vi "field_sweep_agilent.vi"() -> ()   [LabVIEW 2017]
uses:
  Controls/State.ctl
  Controls/Data.ctl
  Controls/Instruments.ctl
  <vilib>/Utility/error.llb/DialogType.ctl
  <vilib>/DAQmx/write.llb/DAQmx Write (Analog DBL 1Chan 1Samp).vi
  <vilib>/DAQmx/create/channels.llb/DAQmx Create Channel (AO-Voltage-Basic).vi
  <vilib>/DAQmx/miscellaneous.llb/DAQmx Fill In Error Info.vi
  <instrlib>/LakeShore 336/Public/Data/Sensor Data (Single Reading).vi
  <instrlib>/Keysight PNA Series/Keysight PNA Series.lvlib
  <instrlib>/LakeShore 336/Lake Shore 336.lvlib
panel:
  in  "Start Over flag":bool
  out "Temp. Contr. Name (out)":refnum<visa-resource-name>
  in  "Temp. Contr. Name (in)":refnum<visa-resource-name>="LakeShore336"
  out "VNA name (out)":refnum<visa-resource-name>
  in  "VNA name (in)":refnum<visa-resource-name>="vna"
  in  "Display Format":i32(ring) items=["Magnitude Linear", "Magnitude Logarithmic", "Phase", "Unwrapped phase", "Imaginary", "Real", "Polar", "Smith Chart", "Smith Admittance", "SWR", "Group Delay", "Kelvin", "Fahrenheit", "Celsius"]
  in  "Data Type":i32(ring) items=["FDATA", "RDATA", "SDATA", "FMEM", "SMEM", "SDIV"]
  in  "Sweep Generation":i32(ring)=1 items=["Stepped", "Analog"]
  in  "Sweep Mode":i32(ring) items=["Chopped", "Alternate"]
  in  "Sweep Type":i32(ring) items=["Linear", "Logarithmic", "Power", "CW", "Segment", "Phase"]
  out "Gaussmeter Name (out)":refnum<visa-resource-name>
  in  "Gaussmeter Name (in)":refnum<visa-resource-name>="Lakeshore_475"
  in  "Clear button":bool
  in  "Hysteresis":bool caption="Hysteresis On/Off"
  out "DAQ channel (out)":tag="DAQ_6363/ao1"
  in  "Averaging Points":i32=10 min=1 max=3201 step=1
  in  "DAQ channel (in)":tag="DAQ_6363/ao1"
  in  "Exit Button":bool
  in  "IF Bandwidth":dbl(ring)=300.0 items=["10 Hz"=10.0, "30 Hz"=30.0, "100 Hz"=100.0, "300 Hz"=300.0, "1 KHz"=1000.0, "3 KHz"=3000.0, "10 KHz"=10000.0, "30 KHz"=30000.0]
  in  "Speed (Oe/sec)":dbl=50.0
  in  "Frequency (Hz)":dbl=4550000000.0 min=10000000.0 max=6000000000.0
  in  "Save Button":bool
  out "Status":string="Initializing..."
  out "Cursor":cluster{"x":dbl, "y":dbl} {"x" format="%.2f"; "y" format="%.5f"}
  out "Error Out":errorcluster={"status"=TRUE, "code"=-1073807346, "source"="VISA Open in Keysight PNA Series.lvlib:Initialize.vi->field_sweep_agilent.vi"}
  in  "Error In (no error)":errorcluster
  out "SpectrumGraph":cluster{"Old Field":dbl[], "Old Signal":dbl[]}[](graph)
  in  "S-parameter":i32(ring) caption="Measurement" items=["S11", "S21"]
  in  "Start Button":bool
  in  "Stop Button":bool
  in  "Output Power (dBm)":dbl=1.0 min=-25.0 max=5.0 step=0.5
  in  "Number of Points":i32=2000 min=1 max=3201 step=1
  in  "Stop H Field (Oe)":dbl=4200.0 min=-6000.0 max=6000.0 format="%#_6f"
  in  "Start H Field (Oe)":dbl=25.0 min=-6000.0 max=6000.0 format="%#_6f"
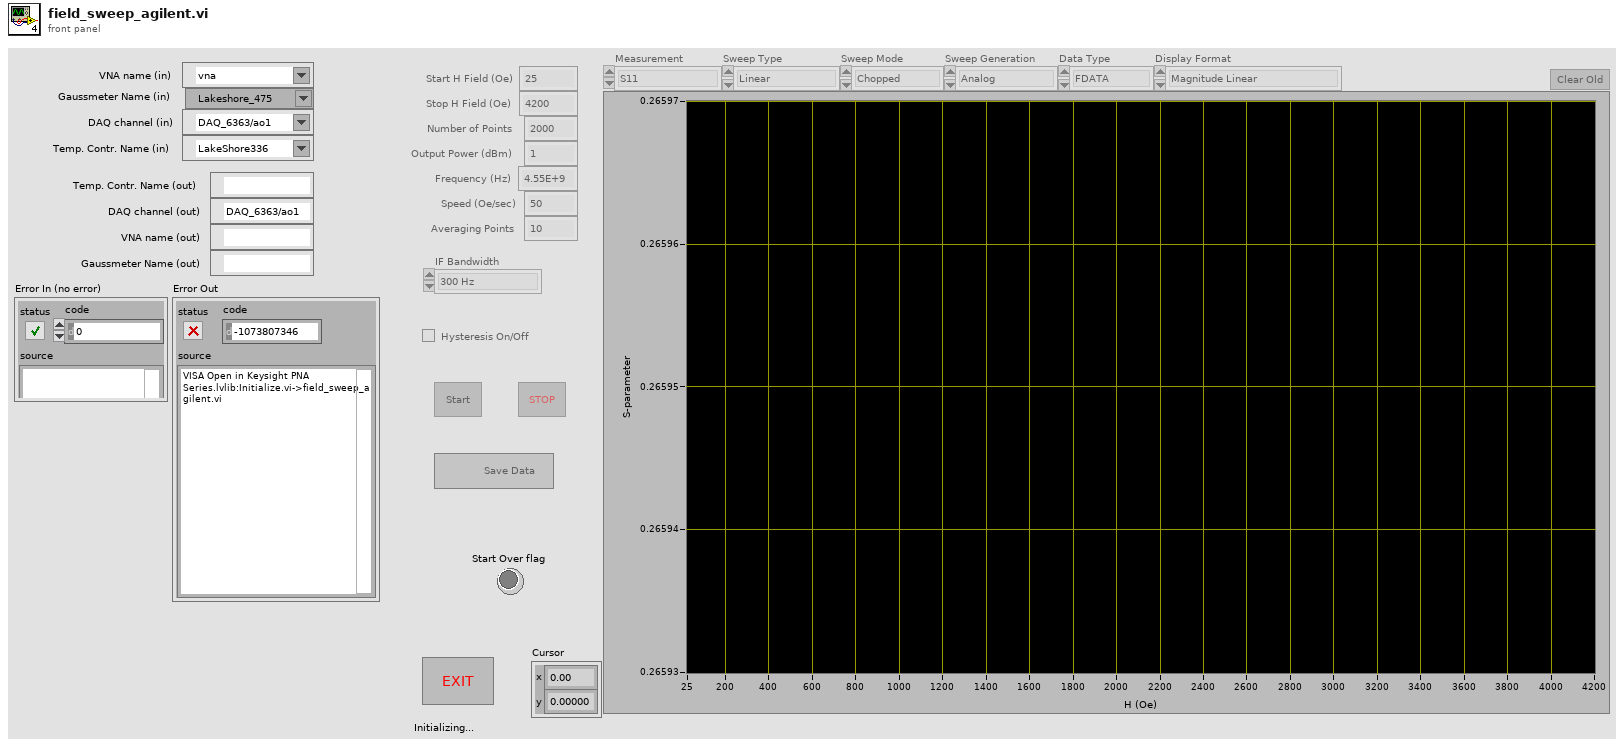
[diagram p1: front panel]
types:
  T1 = typedef "Instruments.ctl" = cluster{"Gaussmeter Name":refnum<visa-resource-name>, "VNA name":refnum<visa-resource-name>, "DAQ channel":tag, "DAQ task":refnum<k21>, "Temp. Contr. Name":refnum<visa-resource-name>}
  T2 = typedef "Data.ctl" = cluster{"Field":dbl[], "Signal":dbl[], "Temperature":dbl[], "Old Field":dbl[], "Old Signal":dbl[], "Old Temperature":dbl[]}
  T3 = typedef "State.ctl" = enum16{"Init", "Idle", "Sweeping up", "Sweeping down", "Running", "Running first time", "Running down", "Shutdown"}
  T4 = cluster{"Baud Rate":u32, "Parity":u16, "Data Bits":u16, "Stop Bits":u16, "Flow Control":u16}
  T5 = typedef "DialogType.ctl" = u16
  T6 = typedef "LVPoint32TypeDef.ctl" = cluster{"Horizontal":i32, "Vertical":i32}
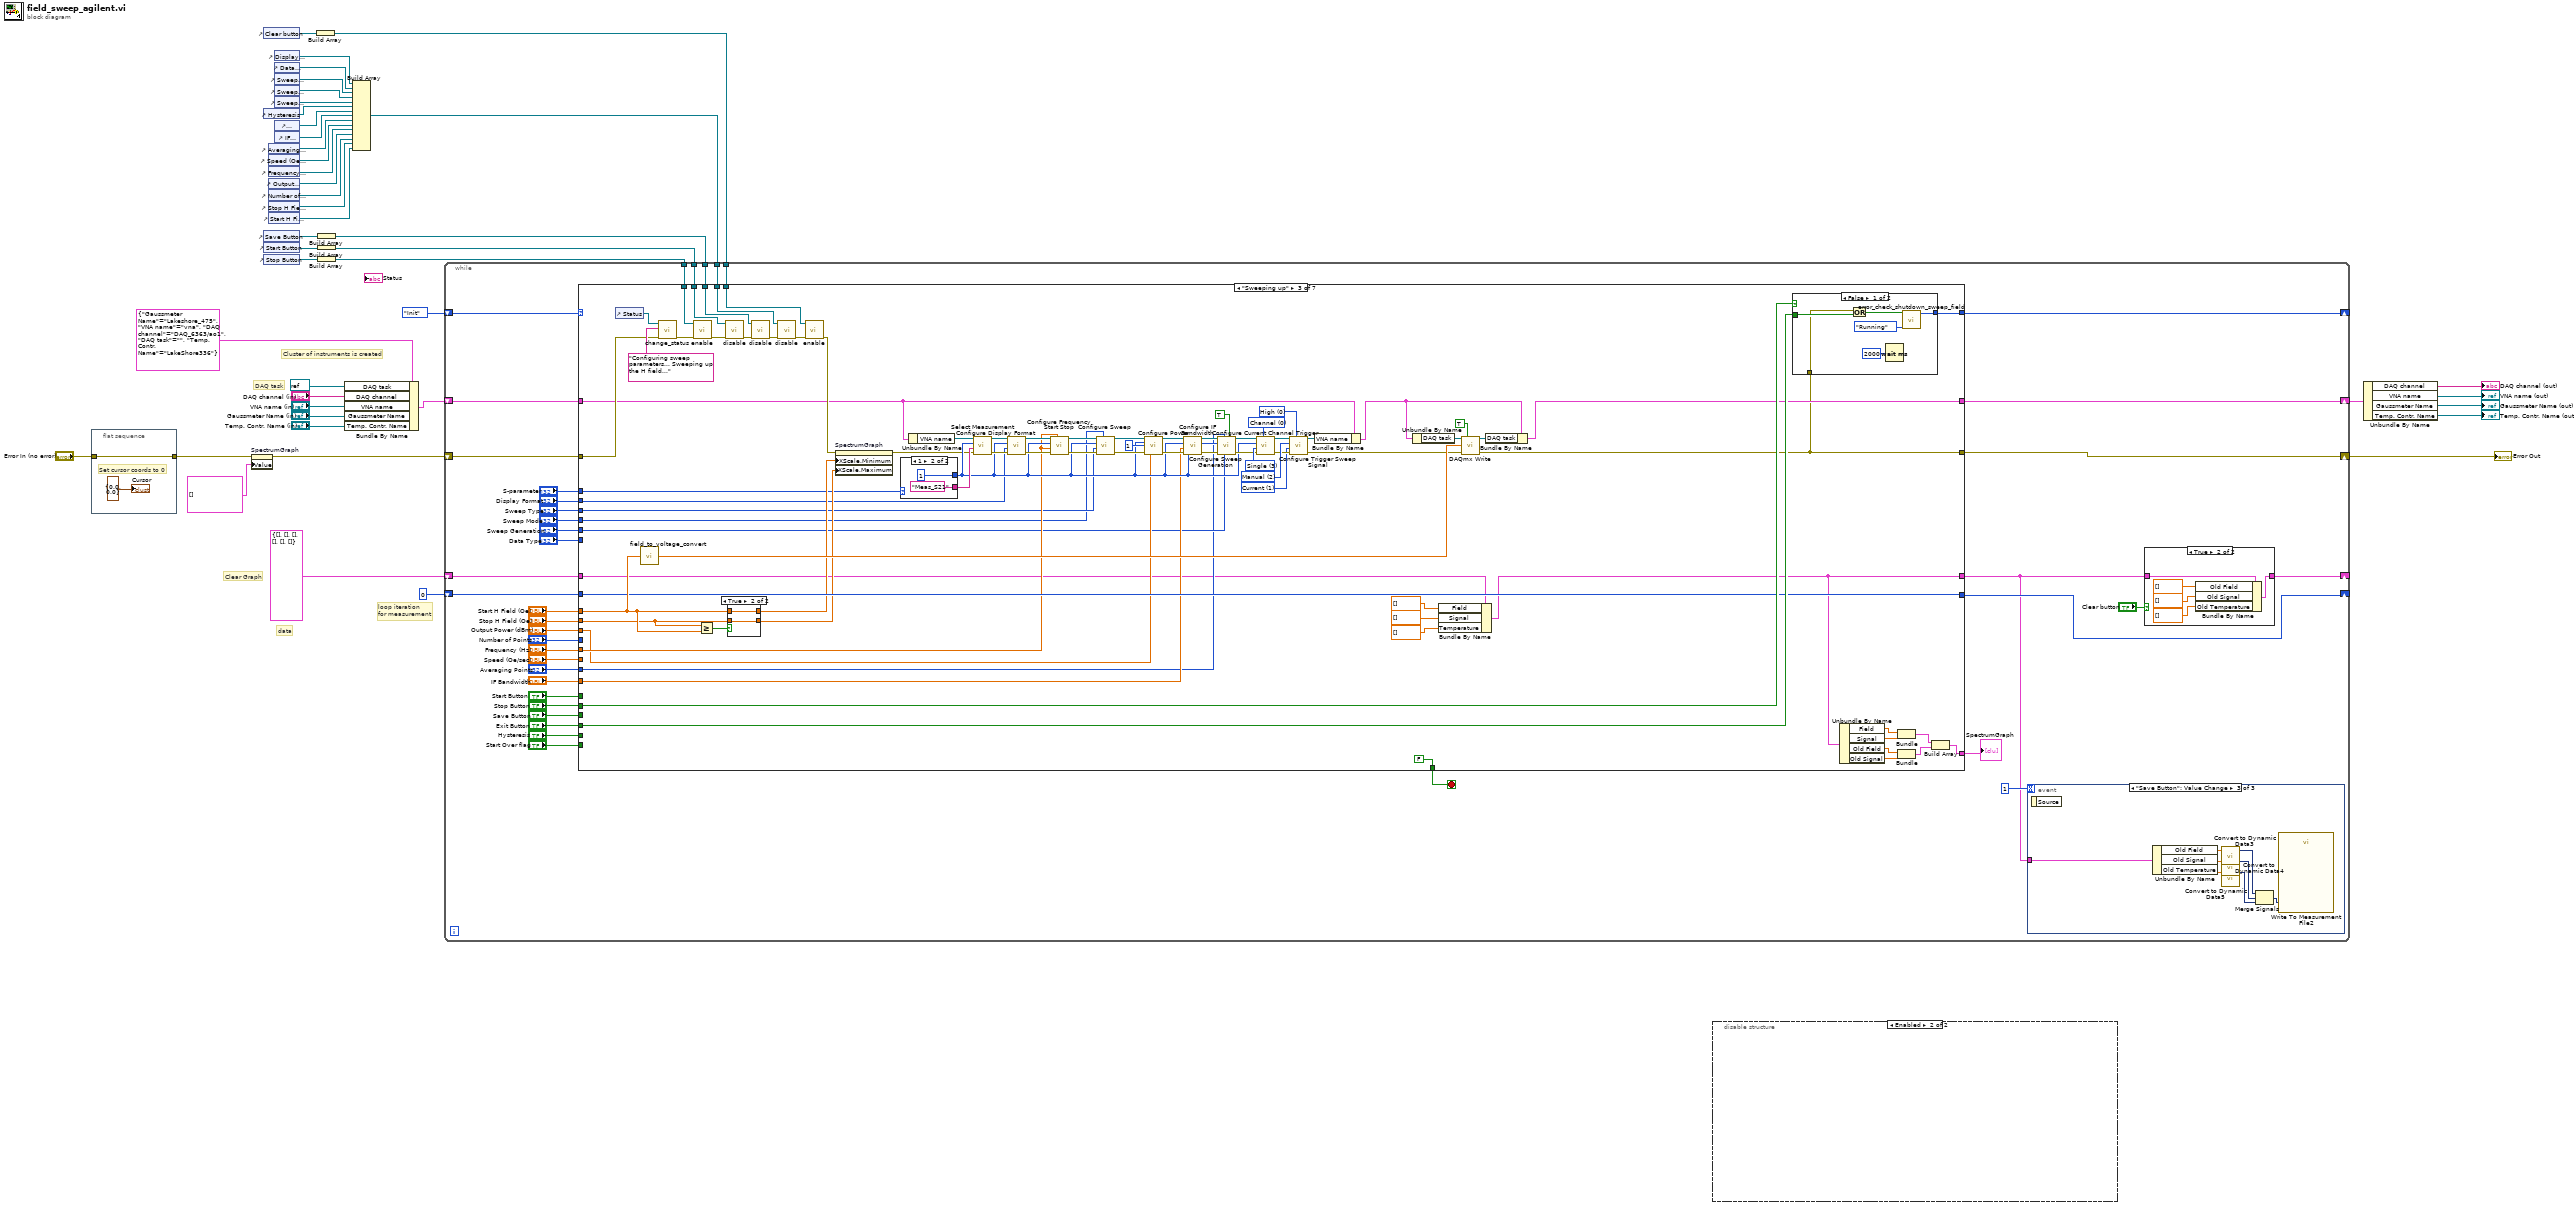
[diagram p0: block diagram]
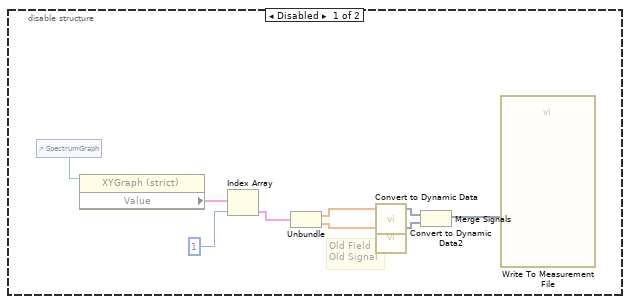
[diagram p2: hidden frame]
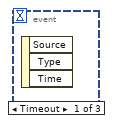
[diagram p4: hidden frame]
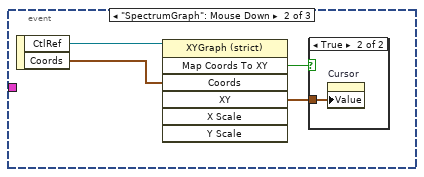
[diagram p5: hidden frame]
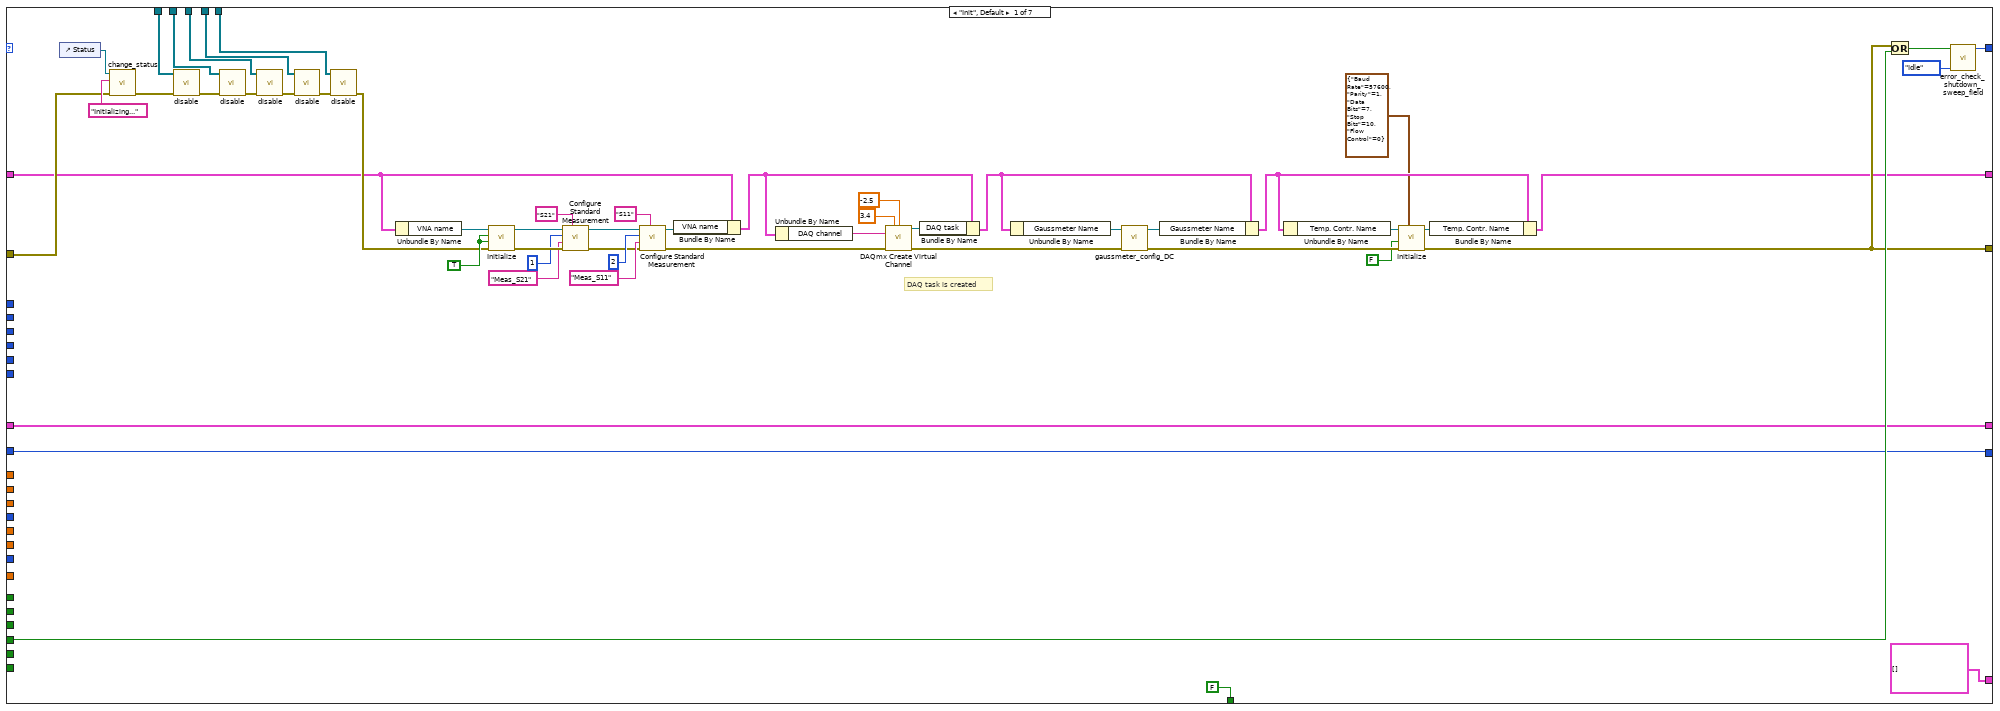
[diagram p7: hidden frame]
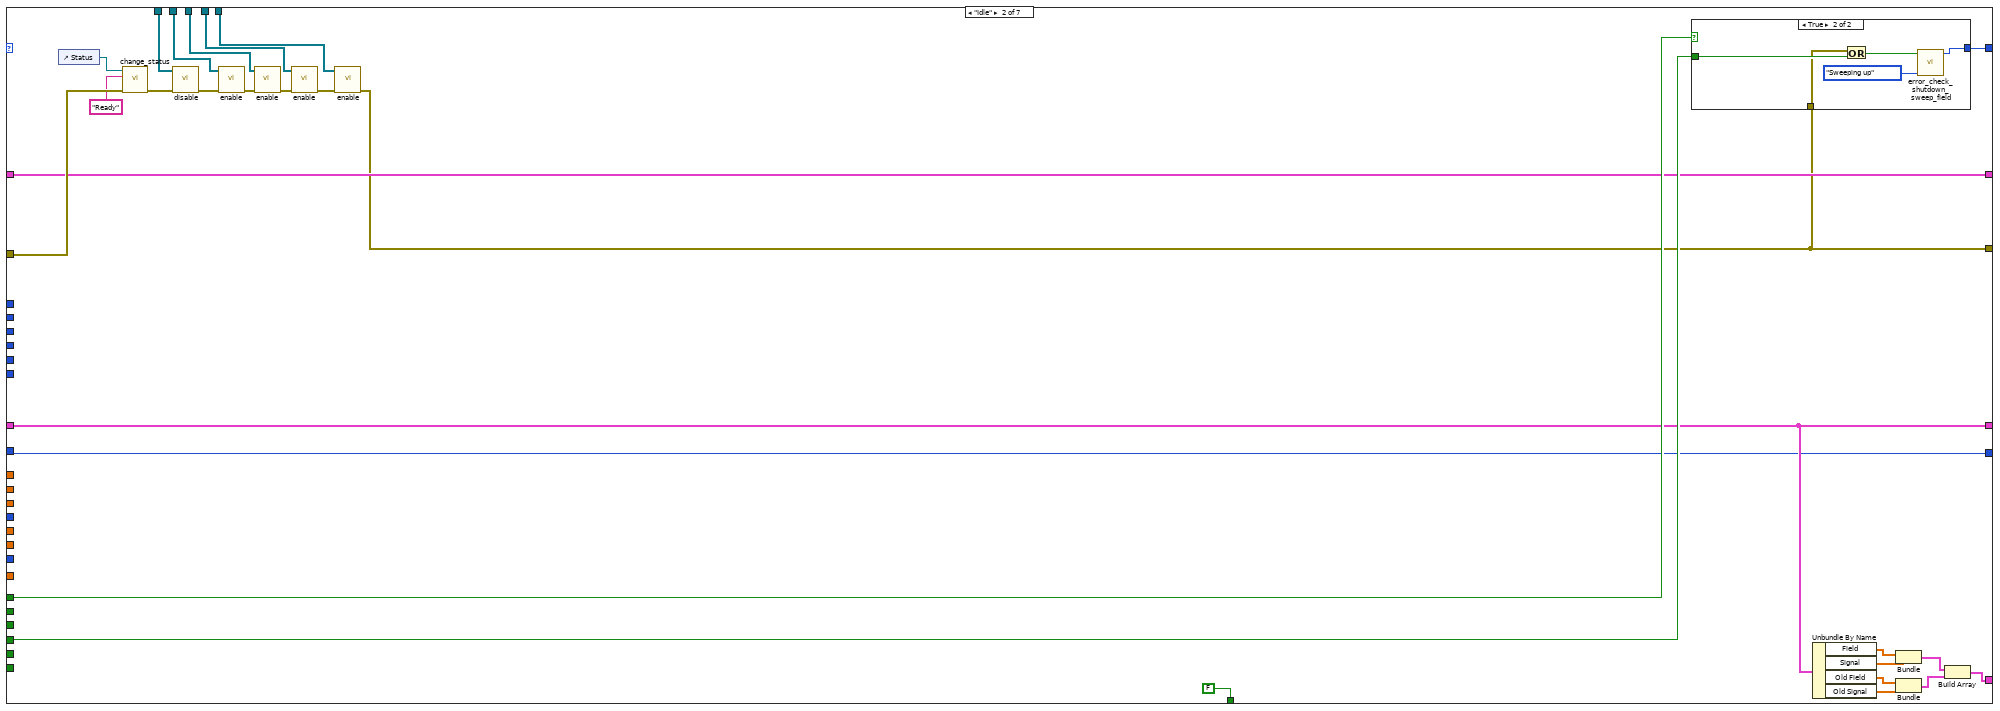
[diagram p8: hidden frame]
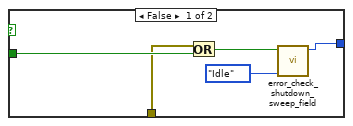
[diagram p9: hidden frame]
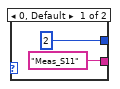
[diagram p10: hidden frame]
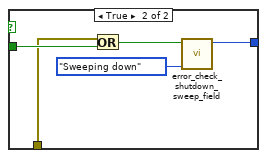
[diagram p12: hidden frame]
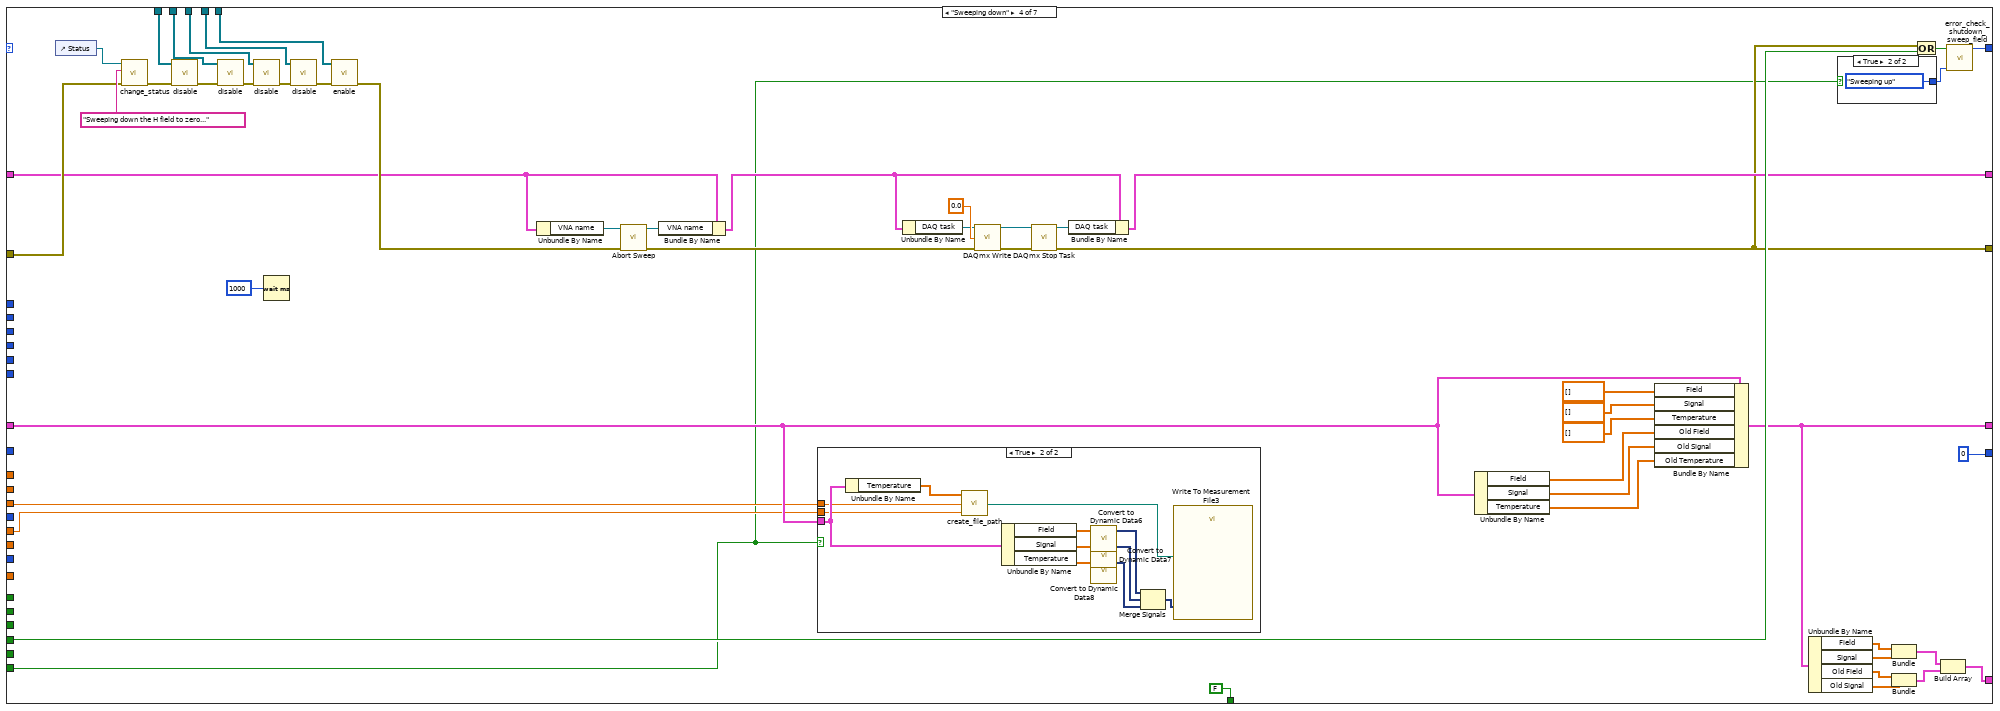
[diagram p13: hidden frame]
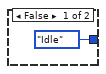
[diagram p15: hidden frame]
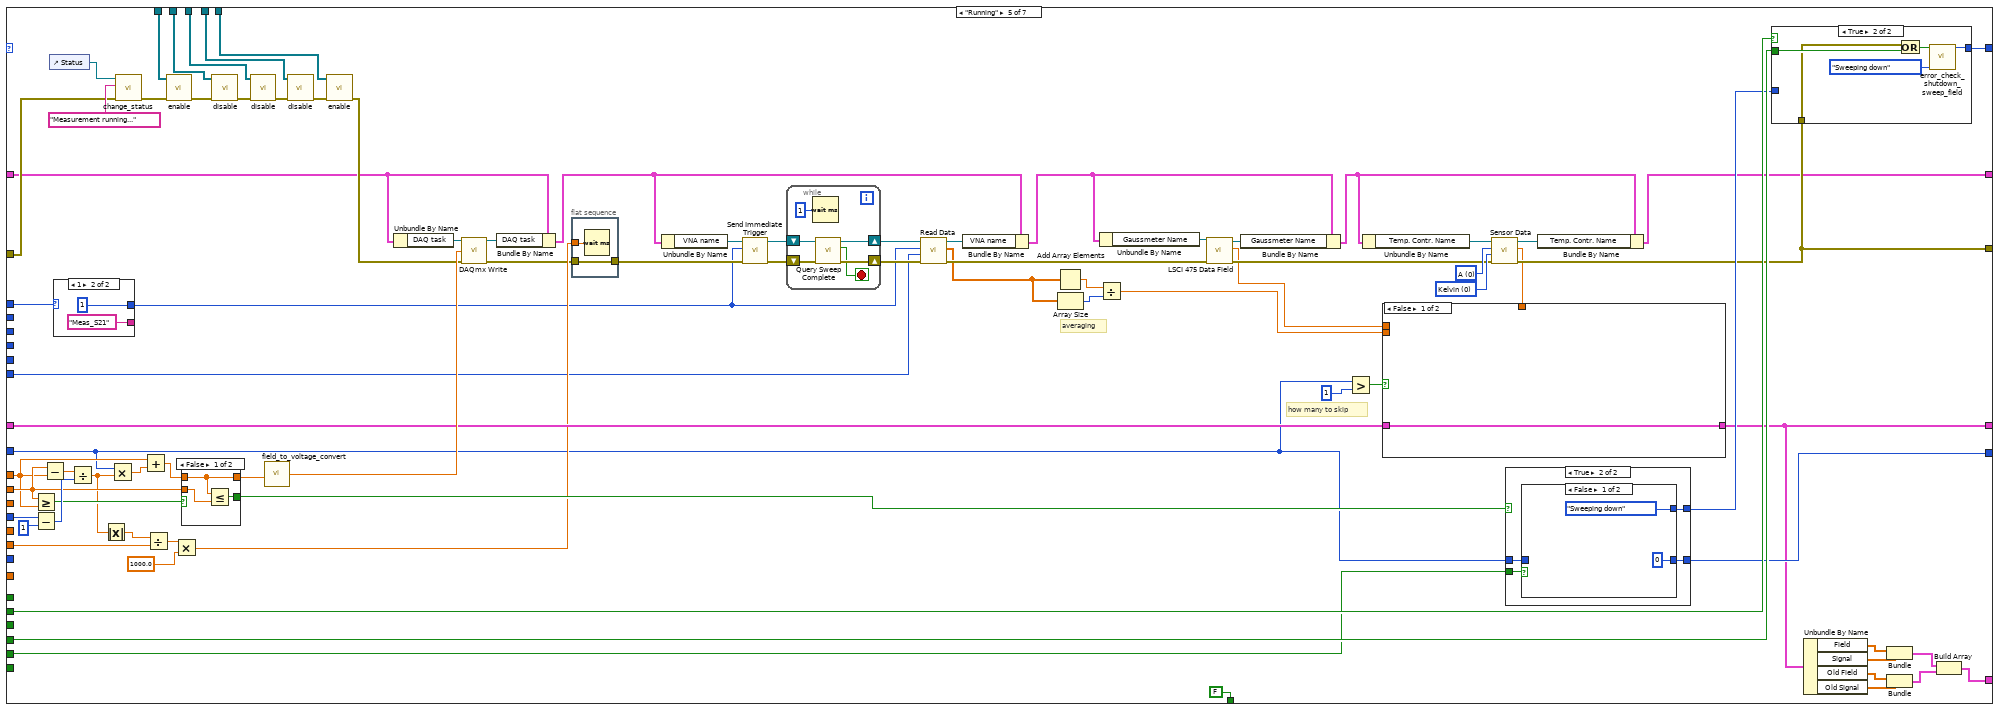
[diagram p16: hidden frame]
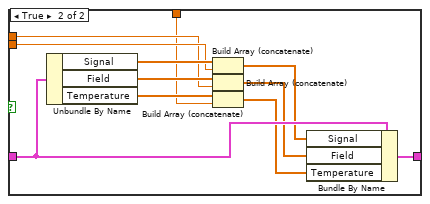
[diagram p17: hidden frame]
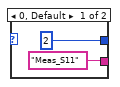
[diagram p18: hidden frame]
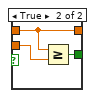
[diagram p19: hidden frame]
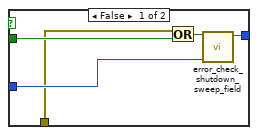
[diagram p20: hidden frame]
diagram:
  # "data"
  # "Cluster of instruments is created"
  # "loop iteration\nfor measurement"
  # "DAQ task"
  # "Clear Graph"
  n1 = flat-sequence {
    tunnel: "Error In (no error)" -> [w45]
    tunnel: [w45] -> w19
    frame #0 {
      # "Set cursor coords to 0"
      "Cursor" <- cluster{"x":dbl, "y":dbl} {"x"=0.0, "y"=0.0} ("Cursor")
    }
  }
  n2 = property on="SpectrumGraph" class="XYGraph (strict)"(error in=w19, "Value"=cluster{"Old Field":dbl[], "Old Signal":dbl[]}[] [] ("SpectrumGraph")) -> (error out=w27:errorcluster)  [unwired: 1 in, 1 out]
  n3 = control-ref of="Clear button"() -> (w22:refnum<vi>)
  n4 = control-ref of="Hysteresis"() -> (w18:refnum<vi>)
  n5 = control-ref of="Save Button"() -> (w31:refnum<vi>)
  n6 = control-ref of="Start Button"() -> (w36:refnum<vi>)
  n7 = control-ref of="Stop Button"() -> (w35:refnum<vi>)
  n8 = control-ref of="Averaging Points"() -> (w28:refnum<vi>)
  n9 = control-ref of="Speed (Oe/sec)"() -> (w42:refnum<vi>)
  n10 = control-ref of="Frequency (Hz)"() -> (w41:refnum<vi>)
  n11 = control-ref of="Output Power (dBm)"() -> (w40:refnum<vi>)
  n12 = control-ref of="Number of Points"() -> (w39:refnum<vi>)
  n13 = control-ref of="Stop H Field (Oe)"() -> (w38:refnum<vi>)
  n14 = control-ref of="Start H Field (Oe)"() -> (w37:refnum<vi>)
  n15 = control-ref of="Display Format"() -> (w13:refnum<vi>)
  n16 = control-ref of="Data Type"() -> (w14:refnum<vi>)
  n17 = control-ref of="Sweep Generation"() -> (w15:refnum<vi>)
  n18 = control-ref of="Sweep Mode"() -> (w16:refnum<vi>)
  n19 = control-ref of="Sweep Type"() -> (w17:refnum<vi>)
  n20 = control-ref of="S-parameter"() -> (w23:refnum<vi>)
  n21 = control-ref of="IF Bandwidth"() -> (w43:refnum<vi>)
  n22 = Build Array(w22) -> (w21:refnum<vi>[])
  n23 = Build Array(w31) -> (w30:refnum<vi>[])
  n24 = Build Array(w36) -> (w33:refnum<vi>[])
  n25 = Build Array(w35) -> (w32:refnum<vi>[])
  n26 = Bundle By Name(cluster=T1 {"Gaussmeter Name"="Lakeshore_475", "VNA name"="vna", "DAQ channel"="DAQ_6363/ao1", "DAQ task"="", "Temp. Contr. Name"="LakeShore336"} ("Cluster"), "DAQ task"=refnum<k21> refnum ("task in"), "DAQ channel"="DAQ channel (in)", "VNA name"="VNA name (in)", "Gaussmeter Name"="Gaussmeter Name (in)", "Temp. Contr. Name"="Temp. Contr. Name (in)") -> (w7:T1)
  n27 = Build Array(w13, w14, w15, w16, w17, w18, w23, w43, w28, w42, w41, w40, w39, w38, w37) -> (w34:refnum<vi>[])
  n28 = while {
    shift-right: [w82] -> _
    shift-left: State."Init" -> [w86]
    shift-right: [w65] -> _
    shift-left: 0 -> [w67]
    tunnel: w34 -> [w85]
    tunnel: w33 -> [w84]
    tunnel: w32 -> [w83]
    shift-right: [w81] -> w24
    shift-left: w27 -> [w80]
    tunnel: w30 -> [w79]
    shift-right: [w57] -> _
    shift-left: T2 {"Field"=[], "Signal"=[], "Temperature"=[], "Old Field"=[], "Old Signal"=[], "Old Temperature"=[]} ("Cluster") -> [w62]
    tunnel: w21 -> [w56]
    shift-right: [w54] -> w6
    shift-left: w7 -> [w55]
    stop <- w74 stop-if-true
    n29 = case shown="\"Sweeping up\"" w86 {
      tunnel: w85 -> [w149 w184 w271 w342 w439 w577 w655]
      tunnel: w84 -> [w157 w186 w273 w340 w441 w579 w657]
      tunnel: w83 -> [w159 w187 w274 w339 w443 w580 w658]
      tunnel: w80 -> [w153 w179 w269 w344 w437 w583 w653]
      tunnel: [w145 w175 w266 w336 w424 w564 State."Shutdown"] -> w82
      tunnel: [w111 w160 w243 w313 w372 w512 w632] -> w81
      tunnel: w79 -> [w150 w185 w272 w341 w440 w578 w656]
      tunnel: "Start Button" -> [_ w176 _ _ _ _ _]
      tunnel: "Stop Button" -> [_ _ w268 _ w427 w572 _]
      tunnel: "Save Button" -> [_ _ _ _ _ _ _]
      tunnel: "Exit Button" -> [w146 w174 w265 w337 w426 w565 _]
      tunnel: [FALSE FALSE FALSE FALSE FALSE FALSE TRUE] -> w74
      tunnel: "Start H Field (Oe)" -> [_ _ w261 _ w403 w555 _]
      tunnel: "Stop H Field (Oe)" -> [_ _ w260 _ w414 w542 _]
      tunnel: "Output Power (dBm)" -> [_ _ w207 w301 _ _ _]
      tunnel: "Number of Points" -> [_ _ _ _ w431 w558 _]
      tunnel: "Frequency (Hz)" -> [_ _ w211 w300 _ _ _]
      tunnel: "Speed (Oe/sec)" -> [_ _ _ _ w432 w548 _]
      tunnel: w67 -> [w143 w162 w250 _ w365 w559 w645]
      tunnel: "Averaging Points" -> [_ _ w204 _ _ _ _]
      tunnel: [w143 w162 w250 0 w400 w540 w645] -> w65
      tunnel: "IF Bandwidth" -> [_ _ w206 _ _ _ _]
      tunnel: [w141 w163 w199 w320 w399 w539 T2 {"Field"=[], "Signal"=[], "Temperature"=[], "Old Field"=[], "Old Signal"=[], "Old Temperature"=[]} ("Cluster")] -> w48
      tunnel: w62 -> [w141 w163 w200 w302 w422 w571 _]
      tunnel: "Hysteresis" -> [_ _ _ _ w412 _ _]
      tunnel: "S-parameter" -> [_ _ w203 _ w391 w521 _]
      tunnel: [cluster{"Old Field":dbl[], "Old Signal":dbl[]}[] [] w166 w253 w321 w411 w554 cluster{"Old Field":dbl[], "Old Signal":dbl[]}[] []] -> w59
      tunnel: w56 -> [w137 w164 w251 w318 w404 w544 w636]
      tunnel: w55 -> [w115 w161 w213 w309 w395 w535 w623]
      tunnel: [w108 w161 w244 w316 w370 w510 w623] -> w54
      tunnel: "Display Format" -> [_ _ w210 _ _ _ _]
      tunnel: "Sweep Type" -> [_ _ w209 _ _ _ _]
      tunnel: "Sweep Mode" -> [_ _ w208 _ _ _ _]
      tunnel: "Sweep Generation" -> [_ _ w205 _ _ _ _]
      tunnel: "Data Type" -> [_ _ _ _ w379 w520 _]
      tunnel: "Start Over flag" -> [_ _ _ w299 _ _ _]
      frame "Init", Default {
        w130 = TRUE ("ID Query (True)")
        # "DAQ task is created"
        n30 = control-ref of="Status"() -> (w155:refnum<vi>)
        n31 = call "change_status.vi"("error in (no error)"=w153, "String"="Initializing...", "String in"=w155) -> ("error out"=w156:errorcluster)  [unwired: 8 in]
        n32 = call "disable.vi"("error in (no error)"=w156, "Array"=w159) -> ("error out"=w158:errorcluster)  [unwired: 9 in]
        n33 = call "disable.vi"("error in (no error)"=w158, "Array"=w157) -> ("error out"=w148:errorcluster)  [unwired: 9 in]
        n34 = call "disable.vi"("error in (no error)"=w148, "Array"=w150) -> ("error out"=w147:errorcluster)  [unwired: 9 in]
        n35 = call "disable.vi"("error in (no error)"=w147, "Array"=w149) -> ("error out"=w138:errorcluster)  [unwired: 9 in]
        n36 = call "disable.vi"("error in (no error)"=w138, "Array"=w137) -> ("error out"=w117:errorcluster)  [unwired: 9 in]
        n37 = Unbundle By Name(w115) -> ("VNA name"=w119:refnum<visa-resource-name>)
        n38 = call <instrlib>:"Initialize.vi"("error in (no error)"=w117, "Reset (True)"=w130, "ID Query (True)"=w130, "VISA resource name"=w119) -> ("error out"=w129:errorcluster, "VISA resource name out"=w128:refnum<visa-resource-name>)  [unwired: 6 in]
        n39 = call <instrlib>:"Configure Standard Measurement.vi"("Measurement Parameters (S11)"="S21", "error in (no error)"=w129, "Measurement Name (CH1_S11_1)"="Meas_S21", "Channel (1)"=1, "VISA resource name"=w128) -> ("error out"=w121:errorcluster, "VISA resource name out"=w120:refnum<visa-resource-name>)  [unwired: 5 in]
        n40 = call <instrlib>:"Configure Standard Measurement.vi"("Measurement Parameters (S11)"="S11", "error in (no error)"=w121, "Measurement Name (CH1_S11_1)"="Meas_S11", "Channel (1)"=2, "VISA resource name"=w120) -> ("error out"=w116:errorcluster, "VISA resource name out"=w118:refnum<visa-resource-name>)  [unwired: 5 in]
        n41 = Bundle By Name(cluster=w115, "VNA name"=w118) -> (w114:T1)
        n42 = Unbundle By Name(w114) -> ("DAQ channel"=w136:tag)
        n43 = call-poly <vilib>:"DAQmx Create Virtual Channel.vi"("maximum value"=3.4, "minimum value"=-2.5, "physical channels"=w136, "error in"=w116) -> ("task out"=w135:refnum<k21>, "error out"=w134:errorcluster)  [unwired: 10 in]
        n44 = Bundle By Name(cluster=w114, "DAQ task"=w135) -> (w131:T1)
        n45 = Unbundle By Name(w131) -> ("Gaussmeter Name"=w133:refnum<visa-resource-name>)
        n46 = call "gaussmeter_config_DC.vi"("error in (no error)"=w134, "VISA Refnum in"=w133) -> ("error out"=w113:errorcluster, "VISA Refnum out"=w132:refnum<visa-resource-name>)  [unwired: 8 in]
        n47 = Bundle By Name(cluster=w131, "Gaussmeter Name"=w132) -> (w109:T1)
        n48 = Unbundle By Name(w109) -> ("Temp. Contr. Name"=w112:refnum<visa-resource-name>)
        n49 = call <instrlib>:"Initialize.vi"("Serial Configuration"=T4 {"Baud Rate"=57600, "Parity"=1, "Data Bits"=7, "Stop Bits"=10, "Flow Control"=0}, "error in (no error)"=w113, "Reset (True)"=FALSE, "VISA resource name"=w112) -> ("error out"=w111:errorcluster, "VISA resource name out"=w110:refnum<visa-resource-name>)  [unwired: 6 in]
        n50 = Bundle By Name(cluster=w109, "Temp. Contr. Name"=w110) -> (w108:T1)
        n51 = Or(x=w111, y=w146) -> (x .or. y?=w144:bool)
        n52 = call "error_check_shutdown_sweep_field.vi"("State In"=State."Idle", "Boolean"=w144) -> ("State Out"=w145:T3)  [unwired: 9 in]
      }
      frame "Idle" {
        n53 = control-ref of="Status"() -> (w178:refnum<vi>)
        n54 = call "change_status.vi"("error in (no error)"=w179, "String"="Ready", "String in"=w178) -> ("error out"=w180:errorcluster)  [unwired: 8 in]
        n55 = call "disable.vi"("error in (no error)"=w180, "Array"=w187) -> ("error out"=w183:errorcluster)  [unwired: 9 in]
        n56 = call "enable.vi"("error in (no error)"=w183, "Array"=w186) -> ("error out"=w182:errorcluster)  [unwired: 9 in]
        n57 = call "enable.vi"("error in (no error)"=w182, "Array"=w185) -> ("error out"=w181:errorcluster)  [unwired: 9 in]
        n58 = call "enable.vi"("error in (no error)"=w181, "Array"=w184) -> ("error out"=w165:errorcluster)  [unwired: 9 in]
        n59 = call "enable.vi"("error in (no error)"=w165, "Array"=w164) -> ("error out"=w160:errorcluster)  [unwired: 9 in]
        n60 = case shown="True" w176 {
          tunnel: [w191 w195] -> w175
          tunnel: w174 -> [w190 w196]
          tunnel: w160 -> [w188 w193]
          frame False {
            n61 = Or(x=w188, y=w190) -> (x .or. y?=w192:bool)
            n62 = call "error_check_shutdown_sweep_field.vi"("State In"=State."Idle", "Boolean"=w192) -> ("State Out"=w191:T3)  [unwired: 9 in]
          }
          frame True {
            n63 = Or(x=w193, y=w196) -> (x .or. y?=w197:bool)
            n64 = call "error_check_shutdown_sweep_field.vi"("State In"=State."Sweeping up", "Boolean"=w197) -> ("State Out"=w195:T3)  [unwired: 9 in]
          }
        }
        n65 = Unbundle By Name(w163) -> ("Field"=w172:dbl[], "Signal"=w171:dbl[], "Old Field"=w170:dbl[], "Old Signal"=w169:dbl[])
        n66 = Bundle("Field"=w172, "Signal"=w171) -> (w168:cluster{"Field":dbl[], "Signal":dbl[]})  [unwired: 1 in]
        n67 = Bundle("Old Field"=w170, "Old Signal"=w169) -> (w167:cluster{"Old Field":dbl[], "Old Signal":dbl[]})  [unwired: 1 in]
        n68 = Build Array(w168, w167) -> (w166:cluster{"Old Field":dbl[], "Old Signal":dbl[]}[])
      }
      frame "Sweeping up" {
        w223 = 0 items=["High", "Low"] ("Trigger Level (1: Low)")
        w224 = 1 items=["All", "Current"] ("Trigger Scope (0: All)")
        w225 = 0 items=["Channel", "Sweep", "Point", "Trace"] ("Trigger Mode (0: Channel)")
        w230 = 3 items=["Hold", "Continuous", "Groups", "Single"] ("Trigger Condition (1: Continuous)")
        w233 = 2 items=["Immediate", "External", "Manual"] ("Trigger Source (0: Immediate)")
        n69 = control-ref of="Status"() -> (w270:refnum<vi>)
        n70 = call "field_to_voltage_convert.vi"("Start H Field (Oe)"=w261) -> ("Numeric"=w267:dbl)
        n71 = call "change_status.vi"("error in (no error)"=w269, "String"="Configuring sweep parameters... Sweeping up the H field...", "String in"=w270) -> ("error out"=w278:errorcluster)  [unwired: 8 in]
        n72 = call "enable.vi"("error in (no error)"=w278, "Array"=w274) -> ("error out"=w277:errorcluster)  [unwired: 9 in]
        n73 = Greater Or Equal?(x=w260, y=w261) -> (x >= y?=w262:bool)
        n74 = call "disable.vi"("error in (no error)"=w277, "Array"=w273) -> ("error out"=w276:errorcluster)  [unwired: 9 in]
        n75 = case shown="True" w262 {
          tunnel: w261 -> [w285 w287]
          tunnel: w260 -> [w284 w286]
          tunnel: [w284 w287] -> w247
          tunnel: [w285 w286] -> w248
          frame False {
          }
          frame True {
          }
        }
        n76 = call "disable.vi"("error in (no error)"=w276, "Array"=w272) -> ("error out"=w275:errorcluster)  [unwired: 9 in]
        n77 = call "disable.vi"("error in (no error)"=w275, "Array"=w271) -> ("error out"=w252:errorcluster)  [unwired: 9 in]
        n78 = call "enable.vi"("error in (no error)"=w252, "Array"=w251) -> ("error out"=w249:errorcluster)  [unwired: 9 in]
        n79 = property on="SpectrumGraph" class="XYGraph (strict)"(error in=w249, "XScale.Minimum"=w247, "XScale.Maximum"=w248) -> (error out=w217:errorcluster)  [unwired: 1 in, 1 out]
        n80 = case shown="1" w203 {
          tunnel: [2 ("Channel (1)") 1 ("Channel (1)")] -> w218
          tunnel: ["Meas_S11" ("Measurement Name (CH1_S11_1)") "Meas_S21" ("Measurement Name (CH1_S11_1)")] -> w242
          frame 0, Default {
          }
          frame 1 {
          }
        }
        n81 = Unbundle By Name(w213) -> ("VNA name"=w215:refnum<visa-resource-name>)
        n82 = call <instrlib>:"Select Measurement.vi"("error in (no error)"=w217, "Measurement Name (CH1_S11_1)"=w242, "Channel (1)"=w218, "VISA resource name"=w215) -> ("error out"=w222:errorcluster, "VISA resource name out"=w221:refnum<visa-resource-name>)  [unwired: 6 in]
        n83 = call <instrlib>:"Configure Display Format.vi"("error in (no error)"=w222, "Display Format (0: Magnitude Linear)"=w210, "Channel (1)"=w218, "VISA resource name"=w221) -> ("error out"=w219:errorcluster, "VISA resource name out"=w220:refnum<visa-resource-name>)  [unwired: 6 in]
        n84 = call <instrlib>:"Configure Frequency Start Stop.vi"("Stop Frequency (2E+6 Hz)"=w211, "error in (no error)"=w219, "Start Frequency (1E+6 Hz)"=w211, "Channel (1)"=w218, "VISA resource name"=w220) -> ("error out"=w232:errorcluster, "VISA resource name out"=w231:refnum<visa-resource-name>)  [unwired: 5 in]
        n85 = call <instrlib>:"Configure Sweep.vi"("Sweep Mode (0: Chopped)"=w208, "error in (no error)"=w232, "Sweep Type (0: Linear)"=w209, "Channel (1)"=w218, "VISA resource name"=w231) -> ("error out"=w241:errorcluster, "VISA resource name out"=w239:refnum<visa-resource-name>)  [unwired: 5 in]
        n86 = call <instrlib>:"Configure Power.vi"("VISA resource name"=w239, "Channel (1)"=w218, "Port (1)"=1, "error in (no error)"=w241, "Power Level (0 dBm)"=w207) -> ("VISA resource name out"=w238:refnum<visa-resource-name>, "error out"=w240:errorcluster)  [unwired: 9 in]
        n87 = call <instrlib>:"Configure IF Bandwidth.vi"("error in (no error)"=w240, "Bandwidth (100000 Hz)"=w206, "Channel (1)"=w218, "VISA resource name"=w238) -> ("error out"=w236:errorcluster, "VISA resource name out"=w237:refnum<visa-resource-name>)  [unwired: 6 in]
        n88 = call <instrlib>:"Configure Sweep Generation.vi"("Auto Sweep or Dwell Time (T: Enable)"=TRUE, "Sweep Generation (1: Analog)"=w205, "Sweep Points (201)"=w204, "error in (no error)"=w236, "Channel (1)"=w218, "VISA resource name"=w237) -> ("error out"=w229:errorcluster, "VISA resource name out"=w227:refnum<visa-resource-name>)  [unwired: 4 in]
        n89 = call <instrlib>:"Configure Current Channel Trigger.vi"("Trigger Mode (0: Channel)"=w225, "error in (no error)"=w229, "Trigger Condition (1: Continuous)"=w230, "Channel (1)"=w218, "VISA resource name"=w227) -> ("error out"=w228:errorcluster, "VISA resource name out"=w226:refnum<visa-resource-name>)  [unwired: 5 in]
        n90 = call <instrlib>:"Configure Trigger Sweep Signal.vi"("Trigger Level (1: Low)"=w223, "error in (no error)"=w228, "Trigger Scope (0: All)"=w224, "Trigger Source (0: Immediate)"=w233, "VISA resource name"=w226) -> ("error out"=w216:errorcluster, "VISA resource name out"=w214:refnum<visa-resource-name>)  [unwired: 5 in]
        n91 = Bundle By Name(cluster=w213, "VNA name"=w214) -> (w212:T1)
        n92 = Unbundle By Name(w212) -> ("DAQ task"=w246:refnum<k21>)
        n93 = Bundle By Name(cluster=w200, "Field"=dbl[] [], "Signal"=dbl[] [], "Temperature"=dbl[] []) -> (w199:T2)
        n94 = call-poly <vilib>:"DAQmx Write.vi"("task/channels in"=w246, "auto start"=TRUE, "data"=w267, "error in"=w216) -> ("task out"=w245:refnum<k21>, "error out"=w243:errorcluster)  [unwired: 9 in, 1 out]
        n95 = Bundle By Name(cluster=w212, "DAQ task"=w245) -> (w244:T1)
        n96 = case shown="False" w268 {
          tunnel: [w292 w297] -> w266
          tunnel: w265 -> [w289 w296]
          tunnel: w243 -> [w288 w294]
          frame False {
            n97 = Or(x=w288, y=w289) -> (x .or. y?=w293:bool)
            n98 = Wait (ms)(milliseconds to wait=u32 2000) -> ()  [unwired: 1 out]
            n99 = call "error_check_shutdown_sweep_field.vi"("State In"=State."Running", "Boolean"=w293) -> ("State Out"=w292:T3)  [unwired: 9 in]
          }
          frame True {
            n100 = Or(x=w294, y=w296) -> (x .or. y?=w298:bool)
            n101 = call "error_check_shutdown_sweep_field.vi"("State In"=State."Sweeping down", "Boolean"=w298) -> ("State Out"=w297:T3)  [unwired: 9 in]
          }
        }
        n102 = Unbundle By Name(w199) -> ("Field"=w259:dbl[], "Signal"=w258:dbl[], "Old Field"=w257:dbl[], "Old Signal"=w256:dbl[])
        n103 = Bundle("Field"=w259, "Signal"=w258) -> (w255:cluster{"Field":dbl[], "Signal":dbl[]})  [unwired: 1 in]
        n104 = Bundle("Old Field"=w257, "Old Signal"=w256) -> (w254:cluster{"Old Field":dbl[], "Old Signal":dbl[]})  [unwired: 1 in]
        n105 = Build Array(w255, w254) -> (w253:cluster{"Old Field":dbl[], "Old Signal":dbl[]}[])
      }
      frame "Sweeping down" {
        n106 = control-ref of="Status"() -> (w335:refnum<vi>)
        n107 = call "change_status.vi"("error in (no error)"=w344, "String"="Sweeping down the H field to zero...", "String in"=w335) -> ("error out"=w348:errorcluster)  [unwired: 8 in]
        n108 = call "disable.vi"("error in (no error)"=w348, "Array"=w339) -> ("error out"=w347:errorcluster)  [unwired: 9 in]
        n109 = call "disable.vi"("error in (no error)"=w347, "Array"=w340) -> ("error out"=w346:errorcluster)  [unwired: 9 in]
        n110 = call "disable.vi"("error in (no error)"=w346, "Array"=w341) -> ("error out"=w345:errorcluster)  [unwired: 9 in]
        n111 = Wait (ms)(milliseconds to wait=u32 1000) -> ()  [unwired: 1 out]
        n112 = call "disable.vi"("error in (no error)"=w345, "Array"=w342) -> ("error out"=w319:errorcluster)  [unwired: 9 in]
        n113 = call "enable.vi"("error in (no error)"=w319, "Array"=w318) -> ("error out"=w312:errorcluster)  [unwired: 9 in]
        n114 = Unbundle By Name(w309) -> ("VNA name"=w311:refnum<visa-resource-name>)
        n115 = call <instrlib>:"Abort Sweep.vi"("error in (no error)"=w312, "VISA resource name"=w311) -> ("error out"=w307:errorcluster, "VISA resource name out"=w310:refnum<visa-resource-name>)  [unwired: 8 in]
        n116 = Bundle By Name(cluster=w309, "VNA name"=w310) -> (w308:T1)
        n117 = case shown="True" w299 {
          tunnel: w302 -> [_ w352]
          tunnel: w301 -> [_ w351]
          tunnel: w300 -> [_ w350]
          frame False {
          }
          frame True {
            n118 = Unbundle By Name(w352) -> ("Temperature"=w354:dbl[])
            n119 = call "create_file_path.vi"("Frequency (Hz)"=w350, "Output Power (dBm)"=w351, "Old Temperature"=w354) -> ("file path"=w353:path)
            n120 = Unbundle By Name(w352) -> ("Field"=w361:dbl[], "Signal"=w359:dbl[], "Temperature"=w355:dbl[])
            n121 = call "Convert to Dynamic Data6"("Array"=w361) -> ("Dynamic Data Type"=w360:dynamicdata)  [unwired: 3 in]
            n122 = call "Convert to Dynamic Data7"("Array"=w359) -> ("Dynamic Data Type"=w358:dynamicdata)  [unwired: 3 in]
            n123 = call "Convert to Dynamic Data8"("Array"=w355) -> ("Dynamic Data Type"=w356:dynamicdata)  [unwired: 3 in]
            n124 = Merge Signals(w360, w358, w356) -> (w357:dynamicdata)
            n125 = call "Write To Measurement File3"("Signals"=w357, "Filename"=w353) -> ()  [unwired: 15 in, 3 out]
          }
        }
        n126 = Unbundle By Name(w308) -> ("DAQ task"=w315:refnum<k21>)
        n127 = call-poly <vilib>:"DAQmx Write.vi"("task/channels in"=w315, "data"=0.0, "error in"=w307) -> ("task out"=w333:refnum<k21>, "error out"=w332:errorcluster)  [unwired: 10 in, 1 out]
        n128 = call <vilib>:"DAQmx Stop Task.vi"("task/channels in"=w333, "error in"=w332) -> ("task out"=w317:refnum<k21>, "error out"=w313:errorcluster)  [unwired: 12 in]
        n129 = Bundle By Name(cluster=w308, "DAQ task"=w317) -> (w316:T1)
        n130 = Unbundle By Name(w302) -> ("Field"=w305:dbl[], "Signal"=w304:dbl[], "Temperature"=w303:dbl[])
        n131 = Bundle By Name(cluster=w302, "Field"=dbl[] [], "Signal"=dbl[] [] ("Field"), "Temperature"=dbl[] [] ("Signal"), "Old Field"=w305, "Old Signal"=w304, "Old Temperature"=w303) -> (w320:T2)
        n132 = Unbundle By Name(w320) -> ("Field"=w327:dbl[], "Signal"=w326:dbl[], "Old Field"=w325:dbl[], "Old Signal"=w324:dbl[])
        n133 = case shown="True" w299 {
          tunnel: [State."Idle" State."Sweeping up"] -> w328
          frame False {
          }
          frame True {
          }
        }
        n134 = Bundle("Field"=w327, "Signal"=w326) -> (w323:cluster{"Field":dbl[], "Signal":dbl[]})  [unwired: 1 in]
        n135 = Bundle("Old Field"=w325, "Old Signal"=w324) -> (w322:cluster{"Old Field":dbl[], "Old Signal":dbl[]})  [unwired: 1 in]
        n136 = Or(x=w313, y=w337) -> (x .or. y?=w338:bool)
        n137 = Build Array(w323, w322) -> (w321:cluster{"Old Field":dbl[], "Old Signal":dbl[]}[])
        n138 = call "error_check_shutdown_sweep_field.vi"("State In"=w328, "Boolean"=w338) -> ("State Out"=w336:T3)  [unwired: 9 in]
      }
      frame "Running" {
        w376 = u16 0 items=["Kelvin", "Celsius", "Sensor Units"] ("Data Source (0:Kelvin)")
        w377 = u16 0 items=["A", "B", "C", "D"] ("Input (0:A)")
        # "how many to skip"
        # "averaging"
        n139 = Greater Or Equal?(x=w414, y=w403) -> (x >= y?=w415:bool)
        n140 = Subtract(x=w431, y=1) -> (x-y=w435:i32)
        n141 = Subtract(x=w414, y=w403) -> (x-y=w429:dbl)
        n142 = control-ref of="Status"() -> (w438:refnum<vi>)
        n143 = case shown="1" w391 {
          tunnel: [2 ("Channel (1)") 1 ("Channel (1)")] -> w380
          tunnel: ["Meas_S11" ("Measurement Name (CH1_S11_1)") "Meas_S21" ("Measurement Name (CH1_S11_1)")] -> _
          frame 0, Default {
          }
          frame 1 {
          }
        }
        n144 = Divide(x=w429, y=w435) -> (x/y=w407:dbl)
        n145 = Absolute Value(x=w407) -> (abs(x)=w406:dbl)
        n146 = Multiply(x=w365, y=w407) -> (x*y=w402:dbl)
        n147 = call "change_status.vi"("error in (no error)"=w437, "String"="Measurement running...", "String in"=w438) -> ("error out"=w444:errorcluster)  [unwired: 8 in]
        n148 = Add(x=w403, y=w402) -> (x+y=w401:dbl)
        n149 = Divide(x=w406, y=w432) -> (x/y=w410:dbl)
        n150 = call "enable.vi"("error in (no error)"=w444, "Array"=w443) -> ("error out"=w447:errorcluster)  [unwired: 9 in]
        n151 = Multiply(x=w410, y=1000.0) -> (x*y=w408:dbl)
        n152 = case shown="False" w415 {
          tunnel: [w470 w473] -> w428
          tunnel: w414 -> [w472 w474]
          tunnel: [w471 w475] -> w413
          tunnel: w401 -> [w470 w473]
          frame False {
            n153 = Less Or Equal?(x=w470, y=w472) -> (x <= y?=w471:bool)
          }
          frame True {
            n154 = Greater Or Equal?(x=w473, y=w474) -> (x >= y?=w475:bool)
          }
        }
        n155 = call "disable.vi"("error in (no error)"=w447, "Array"=w441) -> ("error out"=w446:errorcluster)  [unwired: 9 in]
        n156 = call "disable.vi"("error in (no error)"=w446, "Array"=w440) -> ("error out"=w445:errorcluster)  [unwired: 9 in]
        n157 = call "field_to_voltage_convert.vi"("Start H Field (Oe)"=w428) -> ("Numeric"=w430:dbl)
        n158 = call "disable.vi"("error in (no error)"=w445, "Array"=w439) -> ("error out"=w405:errorcluster)  [unwired: 9 in]
        n159 = call "enable.vi"("error in (no error)"=w405, "Array"=w404) -> ("error out"=w398:errorcluster)  [unwired: 9 in]
        n160 = Unbundle By Name(w395) -> ("DAQ task"=w397:refnum<k21>)
        n161 = call-poly <vilib>:"DAQmx Write.vi"("task/channels in"=w397, "data"=w430, "error in"=w398) -> ("task out"=w396:refnum<k21>, "error out"=w394:errorcluster)  [unwired: 10 in, 1 out]
        n162 = Bundle By Name(cluster=w395, "DAQ task"=w396) -> (w383:T1)
        n163 = flat-sequence {
          tunnel: w408 -> [w500]
          tunnel: w394 -> [w499]
          tunnel: [w499] -> w386
          frame #0 {
            n164 = Wait (ms)(milliseconds to wait=w500) -> ()  [unwired: 1 out]
          }
        }
        n165 = Unbundle By Name(w383) -> ("VNA name"=w381:refnum<visa-resource-name>)
        n166 = call <instrlib>:"Send Immediate Trigger.vi"("error in (no error)"=w386, "Channel (1)"=w380, "VISA resource name"=w381) -> ("error out"=w389:errorcluster, "VISA resource name out"=w390:refnum<visa-resource-name>)  [unwired: 7 in]
        n167 = while {
          shift-right: [w464] -> w388
          shift-left: w389 -> [w465]
          shift-right: [w461] -> w387
          shift-left: w390 -> [w462]
          stop <- w463 stop-if-true
          n168 = Wait (ms)(milliseconds to wait=u32 1) -> ()  [unwired: 1 out]
          n169 = call <instrlib>:"Query Sweep Complete.vi"("error in (no error)"=w465, "VISA resource name"=w462) -> ("error out"=w464:errorcluster, "Sweep Complete"=w463:bool, "VISA resource name out"=w461:refnum<visa-resource-name>)  [unwired: 7 in]
        }
        n170 = call <instrlib>:"Read Data.vi"("error in (no error)"=w388, "Data Type (0: FDATA)"=w379, "Channel (1)"=w380, "VISA resource name"=w387) -> ("error out"=w385:errorcluster, "Data"=w378:dbl[], "VISA resource name out"=w384:refnum<visa-resource-name>)  [unwired: 5 in]
        n171 = Bundle By Name(cluster=w383, "VNA name"=w384) -> (w382:T1)
        n172 = Add Array Elements(numeric array=w378) -> (sum=w434:dbl)
        n173 = Array Size(array=w378) -> (size(s)=w433:i32)
        n174 = Divide(x=w434, y=w433) -> (x/y=w369:dbl)
        n175 = Unbundle By Name(w382) -> ("Gaussmeter Name"=w393:refnum<visa-resource-name>)
        n176 = call <instrlib>:"LSCI 475 Data Field.vi"("error in (no error)"=w385, "VISA session"=w393) -> ("error out"=w373:errorcluster, "Field Reading"=w368:dbl, "dup VISA session"=w392:refnum<visa-resource-name>)  [unwired: 7 in]
        n177 = Bundle By Name(cluster=w382, "Gaussmeter Name"=w392) -> (w371:T1)
        n178 = Greater?(x=w365, y=1) -> (0:w366:bool)
        n179 = Unbundle By Name(w371) -> ("Temp. Contr. Name"=w375:refnum<visa-resource-name>)
        n180 = call-poly <instrlib>:"Sensor Data.vi"("error in (no error)"=w373, "Data Source (0:Kelvin)"=w376, "Input (0:A)"=w377, "VISA resource name"=w375) -> ("error out"=w372:errorcluster, "Sensor Data"=w367:dbl, "VISA resource name out"=w374:refnum<visa-resource-name>)  [unwired: 5 in]
        n181 = case shown="False" w366 {
          tunnel: w422 -> [w448 w459]
          tunnel: [w448 w458] -> w399
          tunnel: w369 -> [_ w454]
          tunnel: w368 -> [_ w453]
          tunnel: w367 -> [_ w452]
          frame False {
          }
          frame True {
            n182 = Unbundle By Name(w459) -> ("Signal"=w457:dbl[], "Field"=w456:dbl[], "Temperature"=w455:dbl[])
            n183 = Build Array (concatenate)(w457, w454) -> (w449:dbl[])
            n184 = Build Array (concatenate)(w456, w453) -> (w450:dbl[])
            n185 = Build Array (concatenate)(w455, w452) -> (w451:dbl[])
            n186 = Bundle By Name(cluster=w459, "Signal"=w449, "Field"=w450, "Temperature"=w451) -> (w458:T2)
          }
        }
        n187 = case shown="True" w413 {
          tunnel: [State."Running" w493] -> w425
          tunnel: w365 -> [w488 w492]
          tunnel: [w486 w490] -> w400
          tunnel: w412 -> [_ w491]
          frame False {
            n188 = Add(x=w488, y=1) -> (x+y=w486:i32)
          }
          frame True {
            n189 = case shown="False" w491 {
              tunnel: [State."Sweeping down" State."Running down"] -> w493
              tunnel: w492 -> [_ _]
              tunnel: [0 0] -> w490
              frame False {
              }
              frame True {
                n190 = Wait (ms)(milliseconds to wait=u32 3000) -> ()  [unwired: 1 out]
              }
            }
          }
        }
        n191 = Bundle By Name(cluster=w371, "Temp. Contr. Name"=w374) -> (w370:T1)
        n192 = case shown="True" w427 {
          tunnel: [w479 w484] -> w424
          tunnel: w426 -> [w478 w483]
          tunnel: w425 -> [w477 _]
          tunnel: w372 -> [w476 w481]
          frame False {
            n193 = Or(x=w476, y=w478) -> (x .or. y?=w480:bool)
            n194 = call "error_check_shutdown_sweep_field.vi"("State In"=w477, "Boolean"=w480) -> ("State Out"=w479:T3)  [unwired: 9 in]
          }
          frame True {
            n195 = Or(x=w481, y=w483) -> (x .or. y?=w485:bool)
            n196 = call "error_check_shutdown_sweep_field.vi"("State In"=State."Sweeping down", "Boolean"=w485) -> ("State Out"=w484:T3)  [unwired: 9 in]
          }
        }
        n197 = Unbundle By Name(w399) -> ("Field"=w421:dbl[], "Signal"=w420:dbl[], "Old Field"=w419:dbl[], "Old Signal"=w418:dbl[])
        n198 = Bundle("Field"=w421, "Signal"=w420) -> (w417:cluster{"Field":dbl[], "Signal":dbl[]})  [unwired: 1 in]
        n199 = Bundle("Old Field"=w419, "Old Signal"=w418) -> (w416:cluster{"Old Field":dbl[], "Old Signal":dbl[]})  [unwired: 1 in]
        n200 = Build Array(w417, w416) -> (w411:cluster{"Old Field":dbl[], "Old Signal":dbl[]}[])
      }
      frame "Running down" {
        w516 = u16 0 items=["Kelvin", "Celsius", "Sensor Units"] ("Data Source (0:Kelvin)")
        w517 = u16 0 items=["A", "B", "C", "D"] ("Input (0:A)")
        # "averaging"
        n201 = Subtract(x=w558, y=1) -> (x-y=w562:i32)
        n202 = Subtract(x=w555, y=w542) -> (x-y=w561:dbl)
        n203 = case shown="1" w521 {
          tunnel: [2 ("Channel (1)") 1 ("Channel (1)")] -> w519
          tunnel: ["Meas_S11" ("Measurement Name (CH1_S11_1)") "Meas_S21" ("Measurement Name (CH1_S11_1)")] -> _
          frame 0, Default {
          }
          frame 1 {
          }
        }
        n204 = control-ref of="Status"() -> (w582:refnum<vi>)
        n205 = Divide(x=w561, y=w562) -> (x/y=w547:dbl)
        n206 = Absolute Value(x=w547) -> (abs(x)=w546:dbl)
        n207 = Multiply(x=w559, y=w547) -> (x*y=w543:dbl)
        n208 = call "change_status.vi"("error in (no error)"=w583, "String"="Measurement running...", "String in"=w582) -> ("error out"=w584:errorcluster)  [unwired: 8 in]
        n209 = Divide(x=w546, y=w548) -> (x/y=w551:dbl)
        n210 = Greater Or Equal?(x=w555, y=w542) -> (x >= y?=w560:bool)
        n211 = Add(x=w543, y=w542) -> (x+y=w541:dbl)
        n212 = Multiply(x=w551, y=1000.0) -> (x*y=w549:dbl)
        n213 = call "enable.vi"("error in (no error)"=w584, "Array"=w580) -> ("error out"=w587:errorcluster)  [unwired: 9 in]
        n214 = case shown="True" w560 {
          tunnel: [w598 w601] -> w556
          tunnel: [w600 w603] -> w557
          tunnel: w555 -> [w599 w602]
          tunnel: w541 -> [w598 w601]
          frame False {
            n215 = Less Or Equal?(x=w598, y=w599) -> (x <= y?=w600:bool)
          }
          frame True {
            n216 = Greater Or Equal?(x=w601, y=w602) -> (x >= y?=w603:bool)
          }
        }
        n217 = call "disable.vi"("error in (no error)"=w587, "Array"=w579) -> ("error out"=w586:errorcluster)  [unwired: 9 in]
        n218 = call "disable.vi"("error in (no error)"=w586, "Array"=w578) -> ("error out"=w585:errorcluster)  [unwired: 9 in]
        n219 = call "disable.vi"("error in (no error)"=w585, "Array"=w577) -> ("error out"=w545:errorcluster)  [unwired: 9 in]
        n220 = call "field_to_voltage_convert.vi"("Start H Field (Oe)"=w556) -> ("Numeric"=w553:dbl)
        n221 = call "enable.vi"("error in (no error)"=w545, "Array"=w544) -> ("error out"=w538:errorcluster)  [unwired: 9 in]
        n222 = Unbundle By Name(w535) -> ("DAQ task"=w537:refnum<k21>)
        n223 = call-poly <vilib>:"DAQmx Write.vi"("task/channels in"=w537, "data"=w553, "error in"=w538) -> ("task out"=w536:refnum<k21>, "error out"=w534:errorcluster)  [unwired: 10 in, 1 out]
        n224 = Bundle By Name(cluster=w535, "DAQ task"=w536) -> (w531:T1)
        n225 = flat-sequence {
          tunnel: w549 -> [w621]
          tunnel: w534 -> [w620]
          tunnel: [w620] -> w525
          frame #0 {
            n226 = Wait (ms)(milliseconds to wait=w621) -> ()  [unwired: 1 out]
          }
        }
        n227 = Unbundle By Name(w531) -> ("VNA name"=w523:refnum<visa-resource-name>)
        n228 = call <instrlib>:"Send Immediate Trigger.vi"("error in (no error)"=w525, "Channel (1)"=w519, "VISA resource name"=w523) -> ("error out"=w528:errorcluster, "VISA resource name out"=w529:refnum<visa-resource-name>)  [unwired: 7 in]
        n229 = while {
          shift-right: [w596] -> w527
          shift-left: w528 -> [w597]
          shift-right: [w593] -> w526
          shift-left: w529 -> [w594]
          stop <- w595 stop-if-true
          n230 = Wait (ms)(milliseconds to wait=u32 1) -> ()  [unwired: 1 out]
          n231 = call <instrlib>:"Query Sweep Complete.vi"("error in (no error)"=w597, "VISA resource name"=w594) -> ("error out"=w596:errorcluster, "Sweep Complete"=w595:bool, "VISA resource name out"=w593:refnum<visa-resource-name>)  [unwired: 7 in]
        }
        n232 = call <instrlib>:"Read Data.vi"("error in (no error)"=w527, "Data Type (0: FDATA)"=w520, "Channel (1)"=w519, "VISA resource name"=w526) -> ("error out"=w524:errorcluster, "Data"=w518:dbl[], "VISA resource name out"=w522:refnum<visa-resource-name>)  [unwired: 5 in]
        n233 = Bundle By Name(cluster=w531, "VNA name"=w522) -> (w530:T1)
        n234 = Add Array Elements(numeric array=w518) -> (sum=w576:dbl)
        n235 = Array Size(array=w518) -> (size(s)=w575:i32)
        n236 = Divide(x=w576, y=w575) -> (x/y=w506:dbl)
        n237 = Unbundle By Name(w530) -> ("Gaussmeter Name"=w533:refnum<visa-resource-name>)
        n238 = call <instrlib>:"LSCI 475 Data Field.vi"("error in (no error)"=w524, "VISA session"=w533) -> ("error out"=w513:errorcluster, "Field Reading"=w505:dbl, "dup VISA session"=w532:refnum<visa-resource-name>)  [unwired: 7 in]
        n239 = Bundle By Name(cluster=w530, "Gaussmeter Name"=w532) -> (w511:T1)
        n240 = Unbundle By Name(w511) -> ("Temp. Contr. Name"=w515:refnum<visa-resource-name>)
        n241 = call-poly <instrlib>:"Sensor Data.vi"("error in (no error)"=w513, "Data Source (0:Kelvin)"=w516, "Input (0:A)"=w517, "VISA resource name"=w515) -> ("error out"=w512:errorcluster, "Sensor Data"=w504:dbl, "VISA resource name out"=w514:refnum<visa-resource-name>)  [unwired: 5 in]
        n242 = Unbundle By Name(w571) -> ("Signal"=w509:dbl[], "Field"=w508:dbl[], "Temperature"=w507:dbl[])
        n243 = Bundle By Name(cluster=w511, "Temp. Contr. Name"=w514) -> (w510:T1)
        n244 = Build Array (concatenate)(w509, w506) -> (w503:dbl[])
        n245 = Build Array (concatenate)(w508, w505) -> (w502:dbl[])
        n246 = Build Array (concatenate)(w507, w504) -> (w501:dbl[])
        n247 = Bundle By Name(cluster=w571, "Signal"=w503, "Field"=w502, "Temperature"=w501) -> (w539:T2)
        n248 = case shown="False" w557 {
          tunnel: [State."Running down" State."Sweeping down"] -> w574
          tunnel: w559 -> [w616 w618]
          tunnel: [w614 w618] -> w540
          frame False {
            n249 = Add(x=w616, y=1) -> (x+y=w614:i32)
          }
          frame True {
          }
        }
        n250 = case shown="True" w572 {
          tunnel: [w607 w612] -> w564
          tunnel: w565 -> [w606 w611]
          tunnel: w574 -> [w605 _]
          tunnel: w512 -> [w604 w609]
          frame False {
            n251 = Or(x=w604, y=w606) -> (x .or. y?=w608:bool)
            n252 = call "error_check_shutdown_sweep_field.vi"("State In"=w605, "Boolean"=w608) -> ("State Out"=w607:T3)  [unwired: 9 in]
          }
          frame True {
            n253 = Or(x=w609, y=w611) -> (x .or. y?=w613:bool)
            n254 = call "error_check_shutdown_sweep_field.vi"("State In"=State."Sweeping down", "Boolean"=w613) -> ("State Out"=w612:T3)  [unwired: 9 in]
          }
        }
        n255 = Unbundle By Name(w539) -> ("Field"=w566:dbl[], "Signal"=w567:dbl[], "Old Field"=w568:dbl[], "Old Signal"=w569:dbl[])
        n256 = Bundle("Field"=w566, "Signal"=w567) -> (w573:cluster{"Field":dbl[], "Signal":dbl[]})  [unwired: 1 in]
        n257 = Bundle("Old Field"=w568, "Old Signal"=w569) -> (w570:cluster{"Old Field":dbl[], "Old Signal":dbl[]})  [unwired: 1 in]
        n258 = Build Array(w573, w570) -> (w554:cluster{"Old Field":dbl[], "Old Signal":dbl[]}[])
      }
      frame "Shutdown" {
        w650 = T5 3 items=["no dialog", "OK message", "continue or stop message", "OK message + warnings", "continue/stop + warnings"] ("type of dialog (OK msg:1)")
        n259 = control-ref of="Status"() -> (w654:refnum<vi>)
        n260 = call "change_status.vi"("error in (no error)"=w653, "String"="Shutting down...Sweeping field to zero...", "String in"=w654) -> ("error out"=w660:errorcluster)  [unwired: 8 in]
        n261 = call "disable.vi"("error in (no error)"=w660, "Array"=w658) -> ("error out"=w663:errorcluster)  [unwired: 9 in]
        n262 = call "disable.vi"("error in (no error)"=w663, "Array"=w657) -> ("error out"=w662:errorcluster)  [unwired: 9 in]
        n263 = call "disable.vi"("error in (no error)"=w662, "Array"=w656) -> ("error out"=w661:errorcluster)  [unwired: 9 in]
        n264 = Wait (ms)(milliseconds to wait=u32 1000) -> ()  [unwired: 1 out]
        n265 = call "disable.vi"("error in (no error)"=w661, "Array"=w655) -> ("error out"=w637:errorcluster)  [unwired: 9 in]
        n266 = call "disable.vi"("error in (no error)"=w637, "Array"=w636) -> ("error out"=w635:errorcluster)  [unwired: 9 in]
        n267 = Unbundle By Name(w623) -> ("DAQ task"=w634:refnum<k21>)
        n268 = call-poly <vilib>:"DAQmx Write.vi"("task/channels in"=w634, "data"=0.0, "error in"=w635) -> ("task out"=w646:refnum<k21>, "error out"=w647:errorcluster)  [unwired: 10 in, 1 out]
        n269 = call <vilib>:"DAQmx Stop Task.vi"("task/channels in"=w646, "error in"=w647) -> ("task out"=w651:refnum<k21>, "error out"=w652:errorcluster)  [unwired: 12 in]
        n270 = call <vilib>:"DAQmx Clear Task.vi"("task in"=w651, "error in"=w652) -> ("error out"=w627:errorcluster)  [unwired: 13 in]
        n271 = Unbundle By Name(w623) -> ("VNA name"=w628:refnum<visa-resource-name>)
        n272 = call <instrlib>:"Abort Sweep.vi"("error in (no error)"=w627, "VISA resource name"=w628) -> ("error out"=w630:errorcluster, "VISA resource name out"=w629:refnum<visa-resource-name>)  [unwired: 8 in]
        n273 = call <instrlib>:"Close.vi"("error in (no error)"=w630, "VISA resource name"=w629) -> ("error out"=w626:errorcluster)  [unwired: 9 in]
        n274 = Unbundle By Name(w623) -> ("Gaussmeter Name"=w631:refnum<visa-resource-name>)
        n275 = call <instrlib>:"LSCI 475 Close.vi"("VISA session"=w631, "error in (no error)"=w626) -> ("error out"=w625:errorcluster)  [unwired: 13 in]
        n276 = Unbundle By Name(w623) -> ("Temp. Contr. Name"=w624:refnum<visa-resource-name>)
        n277 = call <instrlib>:"Close.vi"("error in (no error)"=w625, "VISA resource name"=w624) -> ("error out"=w622:errorcluster)  [unwired: 9 in]
        n278 = property on="SpectrumGraph" class="XYGraph (strict)"(error in=w622, "Value"=cluster{"Old Field":dbl[], "Old Signal":dbl[]}[] [] ("SpectrumGraph")) -> (error out=w642:errorcluster)  [unwired: 1 in, 1 out]
        n279 = control-ref of="Status"() -> (w639:refnum<vi>)
        n280 = call "change_status.vi"("error in (no error)"=w642, "String"="Off", "String in"=w639) -> ("error out"=w641:errorcluster)  [unwired: 8 in]
        n281 = call <vilib>:"Simple Error Handler.vi"("type of dialog (OK msg:1)"=w650, "error in (no error)"=w641) -> ("error out"=w632:errorcluster)  [unwired: 3 in, 4 out]
      }
    }
    "SpectrumGraph" <- w59
    n282 = event shown="[2] \"Save Button\": Value Change" {
      selector: _ -> [_ _ _]
      dyn-events: _ -> [_ _ _]
      timeout: 1 -> [_ _ _]
      tunnel: w48 -> [_ _ w98]
      event Timeout {
        n283 = event-data() -> ()  [unwired: 1 in, 3 out]
      }
      event "SpectrumGraph": Mouse Down {
        n284 = event-data() -> ("CtlRef"=w94:refnum<vi>, "Coords"=w93:T6)  [unwired: 1 in]
        n285 = invoke on="Invoke Node" class="XYGraph (strict)" method="Map Coords To XY"(reference=w94, "Coords"=w93) -> ("Map Coords To XY"=w95:bool, "XY"=w96:cluster{"X":dbl, "Y":dbl})  [unwired: 5 in, 5 out]
        n286 = case shown="True" w95 {
          tunnel: w96 -> [_ w97]
          frame False {
          }
          frame True {
            n287 = property on="Cursor" class="Clust (strict)"("Value"=w97) -> ()  [unwired: 2 in, 2 out]
          }
        }
      }
      event "Save Button": Value Change {
        n288 = event-data() -> ()  [unwired: 1 in, 1 out]
        n289 = Unbundle By Name(w98) -> ("Old Field"=w105:dbl[], "Old Signal"=w103:dbl[], "Old Temperature"=w99:dbl[])
        n290 = call "Convert to Dynamic Data3"("Array"=w105) -> ("Dynamic Data Type"=w104:dynamicdata)  [unwired: 3 in]
        n291 = call "Convert to Dynamic Data4"("Array"=w103) -> ("Dynamic Data Type"=w102:dynamicdata)  [unwired: 3 in]
        n292 = call "Convert to Dynamic Data5"("Array"=w99) -> ("Dynamic Data Type"=w100:dynamicdata)  [unwired: 3 in]
        n293 = Merge Signals(w104, w102, w100) -> (w101:dynamicdata)
        n294 = call "Write To Measurement File2"("Signals"=w101) -> ()  [unwired: 16 in, 3 out]
      }
    }
    n295 = case shown="True" "Clear button" {
      tunnel: w48 -> [w87 w92]
      tunnel: [w87 w91] -> w57
      frame False {
      }
      frame True {
        n296 = Bundle By Name(cluster=w92, "Old Field"=dbl[] [], "Old Signal"=dbl[] [], "Old Temperature"=dbl[] []) -> (w91:T2)
      }
    }
  }
  "Error Out" <- w24
  n297 = disable-structure shown="Enabled" {
    frame Disabled {
      # "Old Field\nOld Signal"
      n298 = control-ref of="SpectrumGraph"() -> (w665:refnum<vi>)
      n299 = property class="XYGraph (strict)"(reference=w665) -> ("Value"=w667:cluster{"Old Field":dbl[], "Old Signal":dbl[]}[])  [unwired: 1 in, 2 out]
      n300 = Index Array(array=w667, index=1) -> (element=w668:cluster{"Old Field":dbl[], "Old Signal":dbl[]})
      n301 = Unbundle(w668) -> ("Old Field"=w672:dbl[], "Old Signal"=w673:dbl[])
      n302 = call "Convert to Dynamic Data"("Array"=w672) -> ("Dynamic Data Type"=w669:dynamicdata)  [unwired: 3 in]
      n303 = call "Convert to Dynamic Data2"("Array"=w673) -> ("Dynamic Data Type"=w670:dynamicdata)  [unwired: 3 in]
      n304 = Merge Signals(w669, w670) -> (w671:dynamicdata)
      n305 = call "Write To Measurement File"("Signals"=w671) -> ()  [unwired: 16 in, 3 out]
    }
    frame Enabled {
    }
  }
  n306 = Unbundle By Name(w6) -> ("DAQ channel"=→"DAQ channel (out)":tag, "VNA name"=→"VNA name (out)":refnum<visa-resource-name>, "Gaussmeter Name"=→"Gaussmeter Name (out)":refnum<visa-resource-name>, "Temp. Contr. Name"=→"Temp. Contr. Name (out)":refnum<visa-resource-name>)
